vi "QTrkSetPixelGainOffset.vi"(8 "error in (no error)":errorcluster, 9 "Gain":sgl[][][](array[numeric]), 10 "Offset":sgl[][][](array[numeric]), 11 "QTrk Instance":T1) -> (0 "error out":errorcluster, 3 "QTrk Instance":T1)   [LabVIEW 2011]
uses:
  QTrkInstance.ctl
  QTrkDLL.vi
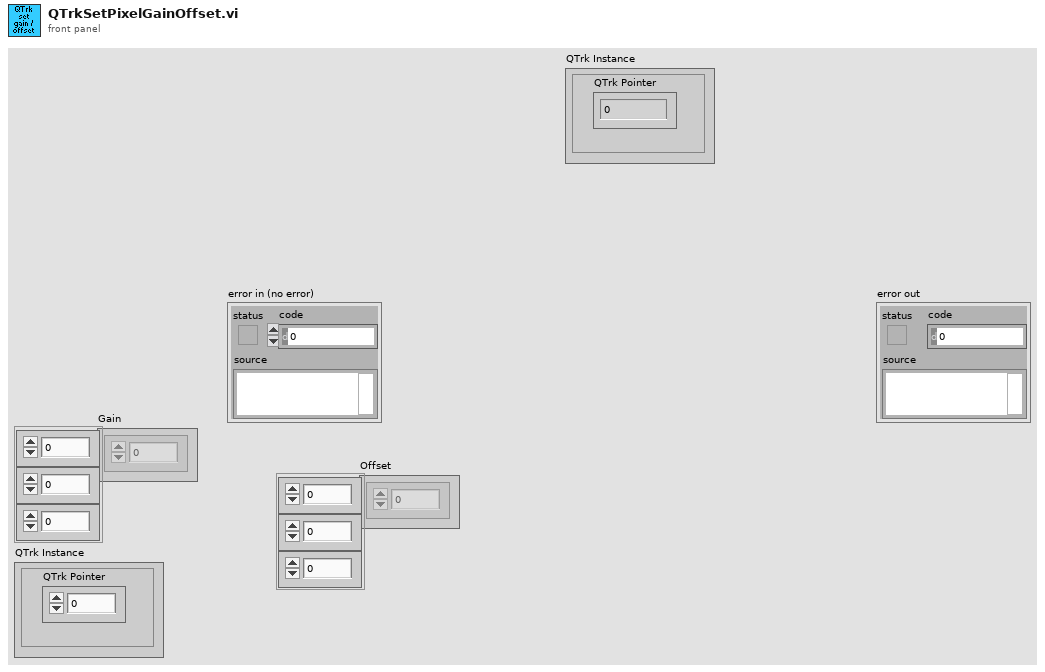
[diagram p1: front panel]
types:
  T1 = typedef "QTrkInstance.ctl" = cluster{"QTrk Pointer":u64}
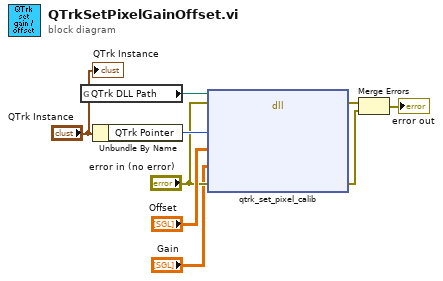
[diagram p0: block diagram]
diagram:
  n1 = global read "QTrkDLL.vi" "QTrk DLL Path"() -> (w7:path)
  n2 = Unbundle By Name("QTrk Instance") -> ("QTrk Pointer"=w9:u64)
  n3 = dll-call lib="D:/jcnossen1/cudaqi-tracker/bin/jtrk-labview.dll" fn="qtrk_set_pixel_calib"(path in=w7, error in="error in (no error)", "tracker"=w9, "offset"="Offset", "gain"="Gain", "error"="error in (no error)") -> (error out=w5:errorcluster, "error"=w4:errorcluster)  [unwired: 5 in, 1 out]
  n4 = Merge Errors(w5, w4) -> (→"error out":errorcluster)
  "QTrk Instance" <- "QTrk Instance"
